vi "wd_length_replaceInIndex.vi"(8 "error in (no error)":errorcluster, 10 "channel index":u32, 11 "meta in":T1={"TargetFile"=path "", "StreamMode"=enum."File", "Append?"=FALSE, "ChunkSize"=0, "TimeColumnMode"=enum."Empty", "TimestampFormat"="", "AbsoluteTime?"=FALSE, "FileAttribute "={"Creator"="", "Title"="", "SheetName"=""}, "Column"=[], "FileRef"=refnum, "MemoryRef"=[], "RecordInfo"=[], " ChannelPreviousInfo"=[], "ChannelFirstRecord"=[], "PredefinedFormattedValueLength"=20, "DiskTemplate"={"XMLRef"=[refnum, refnum, refnum, refnum, refnum, refnum], "ZipPath"=path "", "MetaFile"={"Ref"=refnum, "NextRow"=0, "NextPosition"=0, "Block"=[]}, "TempFolder"=path ""}}) -> (0 "error out":errorcluster, 3 "meta out":T1={"TargetFile"=path "", "StreamMode"=enum."File", "Append?"=FALSE, "ChunkSize"=0, "TimeColumnMode"=enum."Empty", "TimestampFormat"="", "AbsoluteTime?"=FALSE, "FileAttribute "={"Creator"="", "Title"="", "SheetName"=""}, "Column"=[], "FileRef"=refnum, "MemoryRef"=[], "RecordInfo"=[], " ChannelPreviousInfo"=[], "ChannelFirstRecord"=[], "PredefinedFormattedValueLength"=20, "DiskTemplate"={"XMLRef"=[refnum, refnum, refnum, refnum, refnum, refnum], "ZipPath"=path "", "MetaFile"={"Ref"=refnum, "NextRow"=0, "NextPosition"=0, "Block"=[]}, "TempFolder"=path ""}})   [LabVIEW 2020, in "NI_ExcelFile.lvlib"]
uses:
  <vilib>/express/express shared/NI_ExcelFile/NI_ExcelFile.lvlib
  <vilib>/express/express shared/NI_ExcelFile/Ctrls/MainData.ctl
  <vilib>/express/express shared/NI_ExcelFile/Ctrls/StreamMode.ctl
  <vilib>/express/express shared/NI_ExcelFile/Ctrls/TimeColumnMode.ctl
  <vilib>/express/express shared/NI_ExcelFile/Ctrls/FileAttribute.ctl
  <vilib>/express/express shared/NI_ExcelFile/Ctrls/Columns.ctl
  <vilib>/express/express shared/NI_ExcelFile/Ctrls/ColumnInfo.ctl
  <vilib>/express/express shared/NI_ExcelFile/Ctrls/DataType.ctl
  <vilib>/express/express shared/NI_ExcelFile/Ctrls/wd_recordInfo.ctl
  <vilib>/express/express shared/NI_ExcelFile/Ctrls/disk_TemplateFile.ctl
  <vilib>/express/express shared/NI_ExcelFile/Ctrls/meta_file.ctl
  <vilib>/express/express shared/NI_ExcelFile/Ctrls/meta_Block.ctl
  <vilib>/express/express shared/NI_ExcelFile/Ctrls/meta_BlockType.ctl
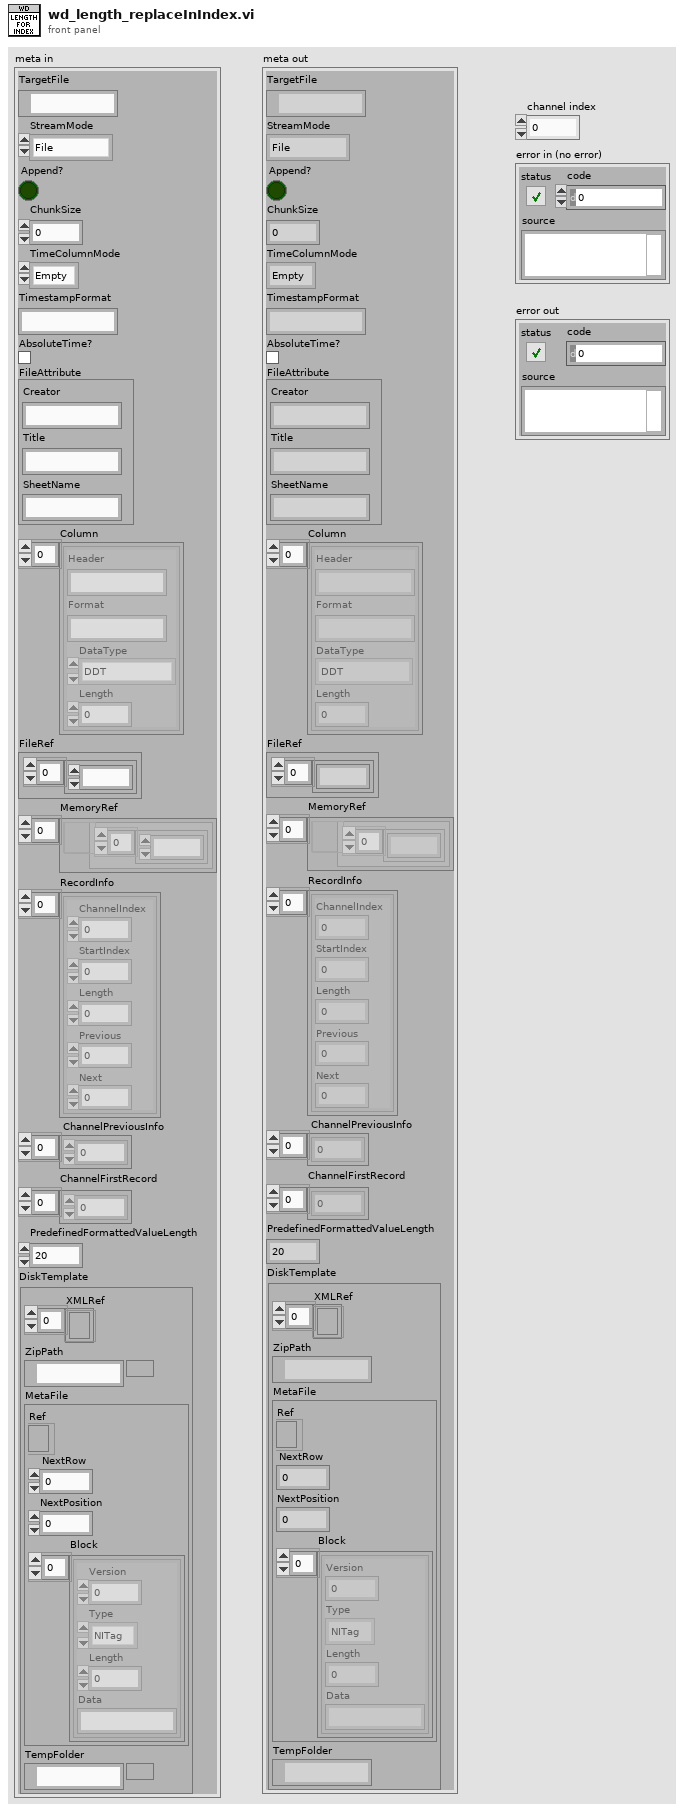
[diagram p1: front panel]
types:
  T1 = typedef "NI_ExcelFile.lvlib/MainData.ctl" = cluster{"TargetFile":path, "StreamMode":T2, "Append?":bool, "ChunkSize":u64, "TimeColumnMode":T3, "TimestampFormat":string, "AbsoluteTime?":bool, "FileAttribute ":T4, "Column":T5, "FileRef":refnum<k1>, "MemoryRef":refnum<data-value>[], "RecordInfo":T8[], " ChannelPreviousInfo":u32[], "ChannelFirstRecord":u32[], "PredefinedFormattedValueLength":i64, "DiskTemplate":T9}
  T2 = typedef "NI_ExcelFile.lvlib/StreamMode.ctl" = enum16{"File", "Memory"}
  T3 = typedef "NI_ExcelFile.lvlib/TimeColumnMode.ctl" = enum16{"Empty", "OnePerCh", "One"}
  T4 = typedef "NI_ExcelFile.lvlib/FileAttribute.ctl" = cluster{"Creator":string, "Title":string, "SheetName":string}
  T5 = typedef "NI_ExcelFile.lvlib/Columns.ctl" = T6[]
  T6 = typedef "NI_ExcelFile.lvlib/ColumnInfo.ctl" = cluster{"Header":string, "Format":string, "DataType":T7, "Length":u64}
  T7 = typedef "NI_ExcelFile.lvlib/DataType.ctl" = enum16{"DDT", "WFM", "Array of STR", "Array of DBL", "Array of I8", "Array of I16", "Array of I32", "Array of I64", "Array of SGL", "Array of U8", "Array of U16", "Array of U32", "Array of U64", "Array of Time"}
  T8 = typedef "NI_ExcelFile.lvlib/wd_recordInfo.ctl" = cluster{"ChannelIndex":u32, "StartIndex":u64, "Length":u64, "Previous":i32, "Next":i32}
  T9 = typedef "NI_ExcelFile.lvlib/disk_TemplateFile.ctl" = cluster{"XMLRef":refnum<file>[], "ZipPath":path, "MetaFile":T10, "TempFolder":path}
  T10 = typedef "NI_ExcelFile.lvlib/meta_file.ctl" = cluster{"Ref":refnum<file>, "NextRow":i32, "NextPosition":i64, "Block":T11[]}
  T11 = typedef "NI_ExcelFile.lvlib/meta_Block.ctl" = cluster{"Version":u16, "Type":T12, "Length":i32, "Data":string}
  T12 = typedef "NI_ExcelFile.lvlib/meta_BlockType.ctl" = enum16{"NITag", "File", "Column"}
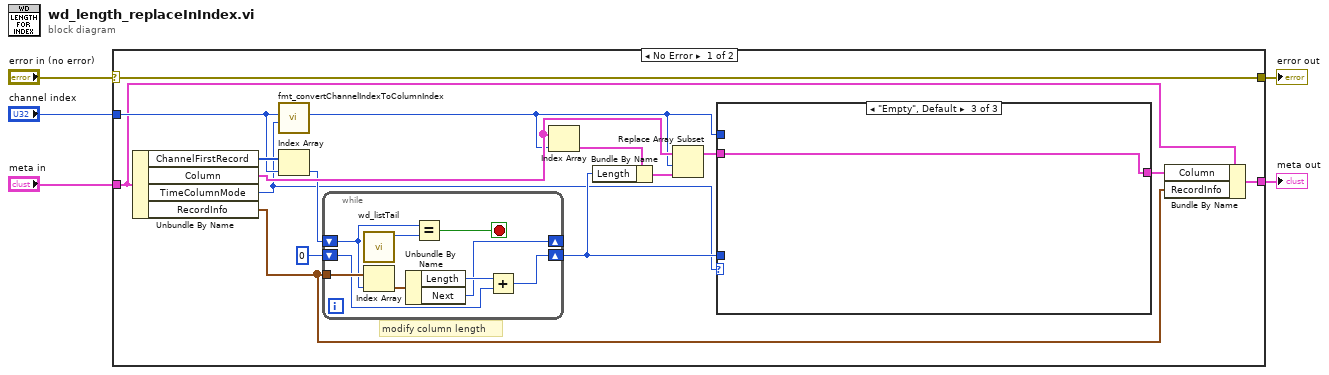
[diagram p0: block diagram]
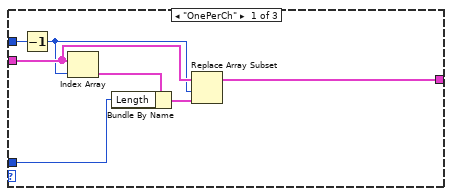
[diagram p2: hidden frame]
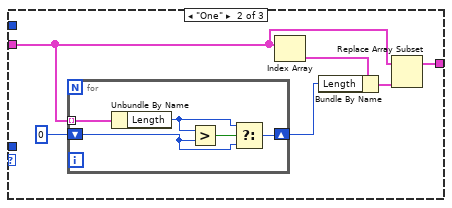
[diagram p3: hidden frame]
diagram:
  n1 = case shown="No Error" "error in (no error)" {
    selector: "error in (no error)" -> [w7 w50]
    tunnel: "channel index" -> [w10 _]
    tunnel: "meta in" -> [w6 w51]
    tunnel: [w19 w51] -> w3
    tunnel: [w7 w50] -> w1
    frame No Error {
      # "modify column length"
      n2 = Unbundle By Name(w6) -> ("ChannelFirstRecord"=w21:u32[], "Column"=w16:T5, "TimeColumnMode"=w9:T3, "RecordInfo"=w11:T8[])
      n3 = call <vilib>:"fmt_convertChannelIndexToColumnIndex.vi"("TimeColumnMode"=w9, "channel index"=w10) -> ("data column index"=w8:i32)  [unwired: 8 in, 1 out]
      n4 = Index Array(array=w21, index=w10) -> (element=w13:u32)
      n5 = while {
        shift-right: [w42] -> _
        shift-left: w13 -> [w48]
        shift-right: [w44] -> w12
        shift-left: 0 -> [w45]
        tunnel: w11 -> [w49]
        stop <- w43 stop-if-true
        n6 = call <vilib>:"wd_listTail.vi"() -> ("list tail"=w41:i32)  [unwired: 11 in]
        n7 = Index Array(array=w49, index=w48) -> (element=w47:T8)
        n8 = Unbundle By Name(w47) -> ("Length"=w46:u64, "Next"=w42:i32)
        n9 = Equal?(x=w48, y=w41) -> (x = y?=w43:bool)
        n10 = Add(x=w46, y=w45) -> (x+y=w44:u64)
      }
      n11 = Index Array(array=w16, index=w8) -> (element=w15:T6)
      n12 = Bundle By Name(cluster=w15, "Length"=w12) -> (w18:T6)
      n13 = Replace Array Subset(array=w16, new element=w18, index=w8) -> (w17:T5)
      n14 = case shown="\"Empty\", Default" w9 {
        tunnel: w17 -> [w24 w31 w40]
        tunnel: [w26 w33 w40] -> w20
        tunnel: w12 -> [w28 _ _]
        tunnel: w8 -> [w27 _ _]
        frame "OnePerCh" {
          n15 = Decrement(x=w27) -> (x-1=w23:i32)
          n16 = Index Array(array=w24, index=w23) -> (element=w22:T6)
          n17 = Bundle By Name(cluster=w22, "Length"=w28) -> (w25:T6)
          n18 = Replace Array Subset(array=w24, new element=w25, index=w23) -> (w26:T5)
        }
        frame "One" {
          n19 = for {
            tunnel: w31 -> [w39] mode=indexing
            shift-right: [w35] -> w29
            shift-left: u64 0 -> [w36]
            n20 = Unbundle By Name(w39) -> ("Length"=w37:u64)
            n21 = Greater?(x=w37, y=w36) -> (0:w38:bool)
            n22 = Select(t=w37, s=w38, f=w36) -> (s? t:f=w35:u64)
          }
          n23 = Index Array(array=w31) -> (element=w32:T6)  [unwired: 1 in]
          n24 = Bundle By Name(cluster=w32, "Length"=w29) -> (w34:T6)
          n25 = Replace Array Subset(array=w31, new element=w34) -> (w33:T5)  [unwired: 1 in]
        }
        frame "Empty", Default {
        }
      }
      n26 = Bundle By Name(cluster=w6, "Column"=w20, "RecordInfo"=w11) -> (w19:T1)
    }
    frame Error {
    }
  }
  "meta out" <- w3
  "error out" <- w1
